vi "Obtain Groups.vi"(10 "Group Configs":refnum<class "Group.lvclass">[](array[class]), 11 "VolatusAPI":refnum<class "VolatusAPI.lvclass">) -> (0 "error out":errorcluster, 2 "Groups":T1[](array[typedef]))   [LabVIEW 2020, in "VolatusDAQGenericGUI.lvlib"]
uses:
  VolatusDAQGenericGUI.lvlib
  Volatus/VolatusAPI/VolatusAPI.lvclass
  VolatusConfig/Group/Group.lvclass
  C:/dev/lv20CE/relink/lv-volatus/VolatusConfig/VolatusConfigElement/VolatusConfigElement.lvclass
  Group Info.ctl
  lv-vecto/Vecto/Group/Group.lvclass
  C:/dev/lv20CE/relink/lv-vecto/Vecto/GroupAbstract/GroupAbstract.lvclass
  VolatusConfig/VolatusConfigElement/VolatusConfigElement.lvclass/VolatusConfigElement.ctl
  lv-vecto/Vecto/GroupAbstract/GroupAbstract.lvclass/GroupAbstract.ctl
  lv-vecto/Vecto/Channel/Channel.lvclass/Channel.ctl
  VolatusConfig/VolatusConfigElement/Element.vi
  lv-vecto/Vecto/GroupAbstract/Channel Info by Index.vi
  VolatusConfig/VolatusConfigElement/VolatusConfigElement.lvclass
  lv-vecto/Vecto/Group Config/Group Config.lvclass
  lv-vecto/Vecto/GroupAbstract/GroupAbstract.lvclass
  lv-vecto/Vecto/Channel/Channel.lvclass
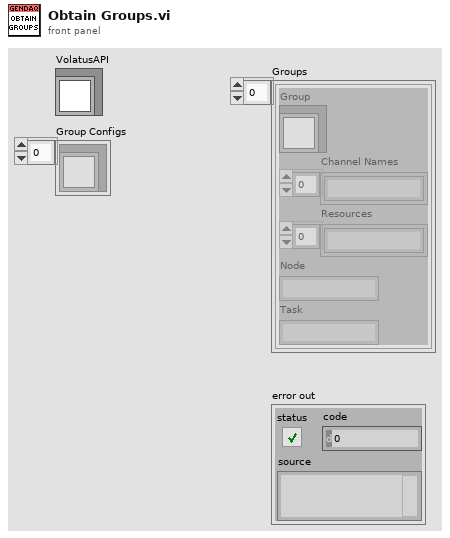
[diagram p1: front panel]
types:
  T1 = typedef "VolatusDAQGenericGUI.lvlib/Group Info.ctl" = cluster{"Group":refnum<class "Group.lvclass">, "Channel Names":string[], "Resources":string[], "Node":string, "Task":string}
  T2 = typedef "VectoConfig.lvlib/Group Info.ctl" = cluster{"System":string, "Cluster":string, "Node":string, "Task":string, "Name":string}
  T3 = typedef "VectoConfig.lvlib/Channel Info.ctl" = cluster{"Name":string, "Group":string, "Owning Node":string, "Owning Task":string, "Resource":string}
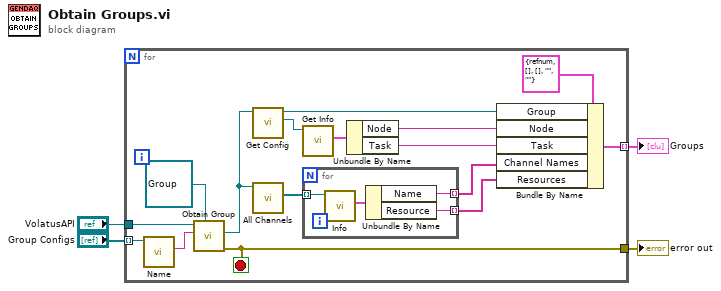
[diagram p0: block diagram]
diagram:
  n1 = for {
    tunnel: "Group Configs" -> [w18] mode=indexing
    tunnel: "VolatusAPI" -> [w20]
    tunnel: [w16] -> w1
    tunnel: [w5] -> w2 mode=indexing
    stop <- w16 stop-if-true
    n2 = call "Name.vi"("VolatusConfigElement in"=w18) -> ("Name"=w17:string)  [unwired: 8 in, 2 out]
    n3 = call "Obtain Group.vi"("Group Type (Abstract)"=refnum<class "Group.lvclass"> refnum ("Vecto.lvlib:Group.lvclass"), "Group Name"=w17, "VolatusAPI in"=w20) -> ("error out"=w16:errorcluster, "Group"=w13:refnum<class "Group.lvclass">)  [unwired: 6 in, 1 out]
    n4 = call "Get Config.vi"("GroupAbstract in"=w13) -> ("Config"=w14:refnum<class "Group Config.lvclass">, "GroupAbstract out"=w6:refnum<class "Group.lvclass">)  [unwired: 8 in, 1 out]
    n5 = call "All Channels.vi"("Group in"=w13) -> ("All Channels"=w12:refnum<class "Channel.lvclass">[])  [unwired: 8 in, 2 out]
    n6 = call "Get Info.vi"("Group Config in"=w14) -> ("Info"=w15:T2)  [unwired: 8 in, 2 out]
    n7 = for {
      tunnel: w12 -> [w23] mode=indexing
      tunnel: [w22] -> w9 mode=indexing
      tunnel: [w21] -> w8 mode=indexing
      n8 = call "Info.vi"("Channel in"=w23) -> ("Info"=w24:T3)  [unwired: 8 in, 2 out]
      n9 = Unbundle By Name(w24) -> ("Name"=w22:string, "Resource"=w21:string)
    }
    n10 = Unbundle By Name(w15) -> ("Node"=w10:string, "Task"=w7:string)
    n11 = Bundle By Name(cluster=T1 {"Group"=refnum, "Channel Names"=[], "Resources"=[], "Node"="", "Task"=""} ("Group Info"), "Group"=w6, "Node"=w10, "Task"=w7, "Channel Names"=w9, "Resources"=w8) -> (w5:T1)
  }
  "Groups" <- w2
  "error out" <- w1
